vi "Interpret Driver Controls.vi"() -> ()   [LabVIEW 2018]
uses:
  SubSystems/Controllers/Manipulator Controlller/Manipulator Controller Global.vi
  SubSystems/Lift/Lift Global.vi
  SubSystems/Controllers/Driver Controller/Driver Controller Global.vi
  SubSystems/Cargo Intake/Cargo Intake Global.vi
  SubSystems/Drive Train/Drive Train Global.vi
  SubSystems/Hatch Panel Intake/Hatch Panel Intake Global.vi
panel:
  in  "y":dbl=0.6 format="%#_13g"
  in  "Y Slower":dbl=0.65
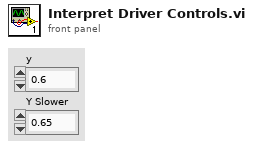
[diagram p1: front panel]
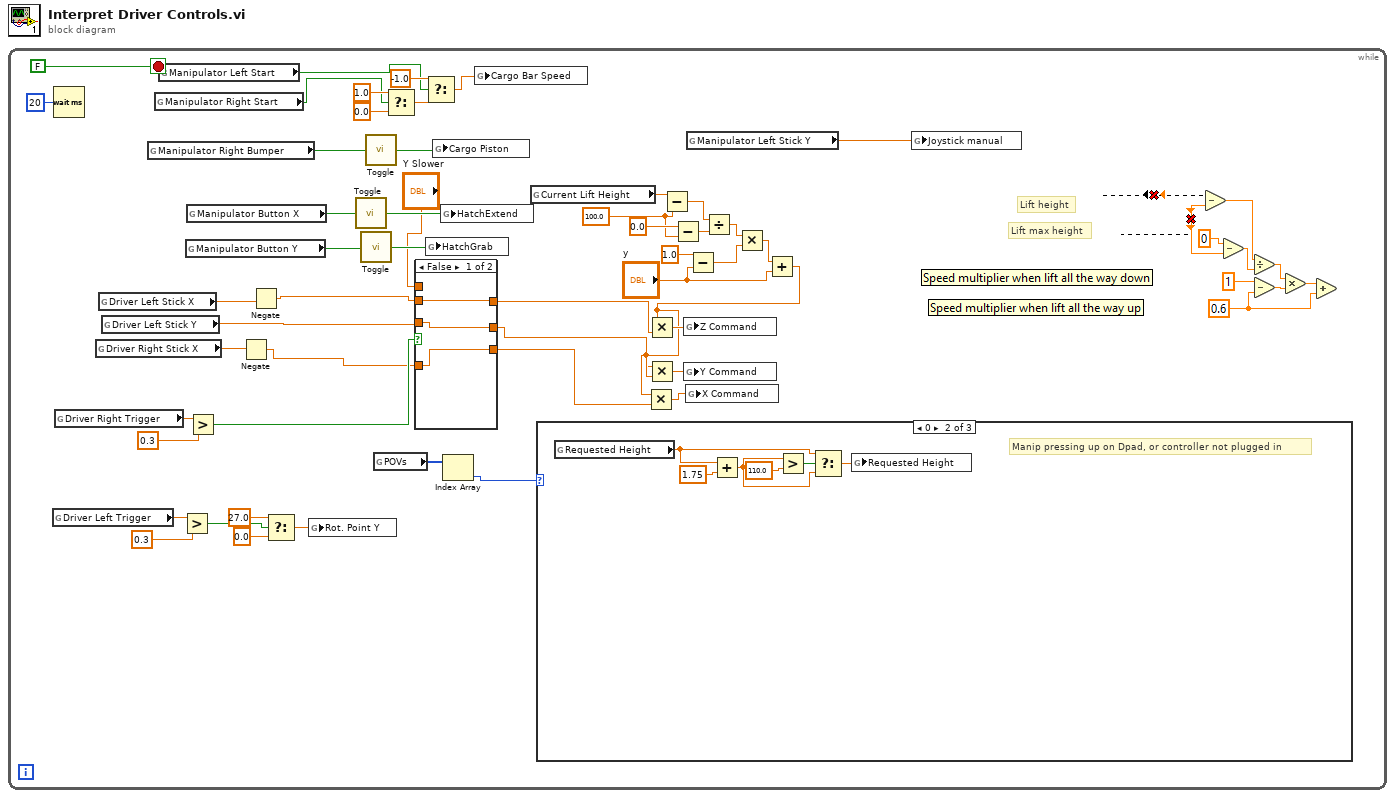
[diagram p0: block diagram]
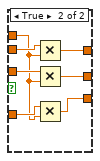
[diagram p2: hidden frame]
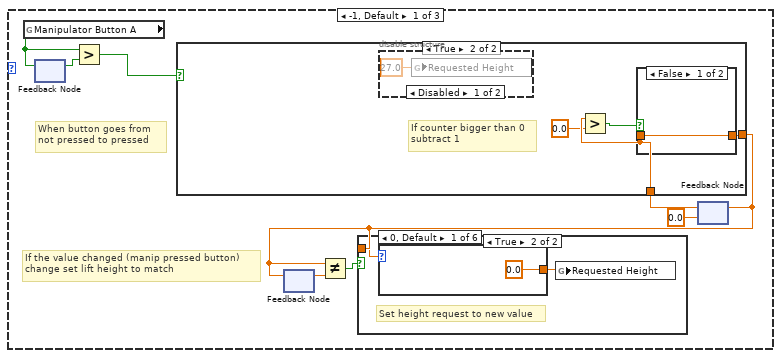
[diagram p3: hidden frame]
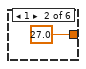
[diagram p5: hidden frame]
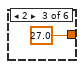
[diagram p6: hidden frame]
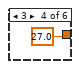
[diagram p7: hidden frame]
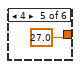
[diagram p8: hidden frame]
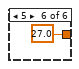
[diagram p9: hidden frame]
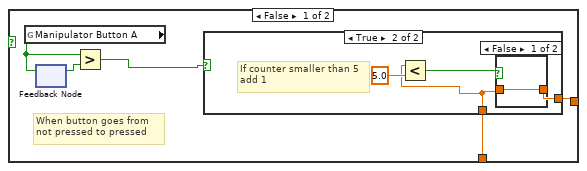
[diagram p10: hidden frame]
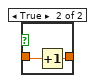
[diagram p12: hidden frame]
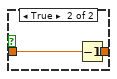
[diagram p13: hidden frame]
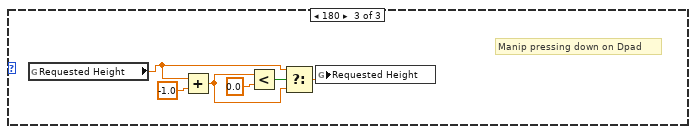
[diagram p15: hidden frame]
diagram:
  n1 = while {
    stop <- FALSE stop-if-true
    w10 = 100.0 ("y")
    # "Lift max height"
    # "Lift height"
    n2 = global read "Driver Controller Global.vi" "Driver Left Trigger"() -> (w5:dbl)
    n3 = Wait (ms)(milliseconds to wait=u32 20) -> ()  [unwired: 1 out]
    n4 = global read "Driver Controller Global.vi" "Driver Right Trigger"() -> (w32:dbl)
    n5 = global read "Driver Controller Global.vi" "Driver Right Stick X"() -> (w38:dbl)
    n6 = global read "Driver Controller Global.vi" "Driver Left Stick X"() -> (w39:dbl)
    n7 = global read "Driver Controller Global.vi" "Driver Left Stick Y"() -> (w8:dbl)
    n8 = global read "Manipulator Controller Global.vi" "Manipulator Right Bumper"() -> (w33:bool)
    n9 = global read "Manipulator Controller Global.vi" "Manipulator Right Start"() -> (w41:bool)
    n10 = global read "Manipulator Controller Global.vi" "Manipulator Left Start"() -> (w42:bool)
    n11 = Greater?(x=w5, y=0.3) -> (0:w3:bool)
    n12 = global read "Manipulator Controller Global.vi" "Manipulator Button Y"() -> (w37:bool)
    n13 = global read "Manipulator Controller Global.vi" "Manipulator Button X"() -> (w48:bool)
    n14 = Greater?(x=w32, y=0.3) -> (0:w28:bool)
    n15 = Negate(x=w38) -> (-x=w7:dbl)
    n16 = Negate(x=w39) -> (-x=w9:dbl)
    n17 = Select(t=27.0, s=w3, f=0.0) -> (s? t:f=w4:dbl)
    n18 = global write "Drive Train Global.vi" "Rot. Point Y"(w4) -> ()
    n19 = call "Toggle.vi"("Input"=w48) -> ("Output"=w47:bool)
    n20 = call "Toggle.vi"("Input"=w37) -> ("Output"=w36:bool)
    n21 = call "Toggle.vi"("Input"=w33) -> ("Output"=w34:bool)
    n22 = global read "Manipulator Controller Global.vi" "POVs"() -> (w30:i16[])
    n23 = Select(t=1.0, s=w41, f=0.0) -> (s? t:f=w46:dbl)
    n24 = case shown="False" w28 {
      tunnel: w9 -> [w53 w60]
      tunnel: "Y Slower" -> [_ w54]
      tunnel: [w53 w59] -> w23
      tunnel: [w52 w58] -> w22
      tunnel: [w51 w57] -> w21
      tunnel: w8 -> [w52 w56]
      tunnel: w7 -> [w51 w55]
      frame False {
      }
      frame True {
        n25 = Multiply(x=w60, y=w54) -> (x*y=w59:dbl)
        n26 = Multiply(x=w56, y=w54) -> (x*y=w58:dbl)
        n27 = Multiply(x=w55, y=w54) -> (x*y=w57:dbl)
      }
    }
    n28 = Select(t=-1.0, s=w42, f=w46) -> (s? t:f=w40:dbl)
    n29 = global write "Hatch Panel Intake Global.vi" "HatchGrab"(w36) -> ()
    n30 = global write "Cargo Intake Global.vi" "Cargo Piston"(w34) -> ()
    n31 = global write "Hatch Panel Intake Global.vi" "HatchExtend"(w47) -> ()
    n32 = Index Array(array=w30) -> (element=w29:i16)  [unwired: 1 in]
    n33 = global write "Cargo Intake Global.vi" "Cargo Bar Speed"(w40) -> ()
    n34 = global read "Lift Global.vi" "Current Lift Height"() -> (w20:dbl)
    n35 = case shown="0" w29 {
      frame -1, Default {
        # "If the value changed (manip pressed button)\nchange set lift height to match"
        # "When button goes from\nnot pressed to pressed"
        n36 = global read "Manipulator Controller Global.vi" "Manipulator Button A"() -> (w67:bool)
        n37 = feedback #1() -> (w68:bool)  [unwired: 1 in]
        n38 = feedback-in #1(w67) -> ()
        n39 = Greater?(x=w67, y=w68) -> (0:w61:bool)
        n40 = feedback #2() -> (w64:dbl)  [unwired: 1 in]
        n41 = feedback #3(0.0) -> (w66:dbl)
        n42 = case shown="True" w61 {
          tunnel: [w78 w93] -> w63
          tunnel: w66 -> [w79 w92]
          frame False {
            # "When button goes from\nnot pressed to pressed"
            n43 = global read "Manipulator Controller Global.vi" "Manipulator Button A"() -> (w81:bool)
            n44 = feedback #4() -> (w80:bool)  [unwired: 1 in]
            n45 = feedback-in #4(w81) -> ()
            n46 = Greater?(x=w81, y=w80) -> (0:w77:bool)
            n47 = case shown="True" w77 {
              tunnel: w79 -> [w82 w84]
              tunnel: [w82 w86] -> w78
              frame False {
              }
              frame True {
                # "If counter smaller than 5\nadd 1"
                n48 = Less?(x=w84, y=5.0) -> (x < y?=w83:bool)
                n49 = case shown="False" w83 {
                  tunnel: [w87 w89] -> w86
                  tunnel: w84 -> [w87 w88]
                  frame False {
                  }
                  frame True {
                    n50 = Increment(x=w88) -> (x+1=w89:dbl)
                  }
                }
              }
            }
          }
          frame True {
            # "If counter bigger than 0\nsubtract 1"
            n51 = disable-structure shown="Disabled" {
              frame Disabled {
                n52 = global write "Lift Global.vi" "Requested Height"(27.0 ("Requested Height")) -> ()
              }
              frame Enabled {
              }
            }
            n53 = Greater?(x=w92, y=0.0) -> (0:w91:bool)
            n54 = case shown="False" w91 {
              tunnel: [w94 w96] -> w93
              tunnel: w92 -> [w94 w95]
              frame False {
              }
              frame True {
                n55 = Decrement(x=w95) -> (x-1=w96:dbl)
              }
            }
          }
        }
        n56 = feedback-in #2(w63) -> ()
        n57 = Not Equal?(x=w63, y=w64) -> (x != y?=w62:bool)
        n58 = case shown="True" w62 {
          tunnel: w63 -> [_ w69]
          frame False {
            # "Manipulator didnt request change"
          }
          frame True {
            # "Set height request to new value"
            n59 = case shown="0, Default" w69 {
              tunnel: [0.0 ("Requested Height") 27.0 ("Requested Height") 27.0 ("Requested Height") 27.0 ("Requested Height") 27.0 ("Requested Height") 27.0 ("Requested Height")] -> w70
              frame 0, Default {
              }
              frame 1 {
              }
              frame 2 {
              }
              frame 3 {
              }
              frame 4 {
              }
              frame 5 {
              }
            }
            n60 = global write "Lift Global.vi" "Requested Height"(w70) -> ()
          }
        }
        n61 = feedback-in #3(w63) -> ()
      }
      frame 0 {
        # "Manip pressing up on Dpad, or controller not plugged in"
        n62 = global read "Lift Global.vi" "Requested Height"() -> (w99:dbl)
        n63 = Add(x=w99, y=1.75) -> (x+y=w98:dbl)
        n64 = Greater?(x=w98, y=110.0) -> (0:w100:bool)
        n65 = Select(t=w99, s=w100, f=w98) -> (s? t:f=w101:dbl)
        n66 = global write "Lift Global.vi" "Requested Height"(w101) -> ()
      }
      frame 180 {
        # "Manip pressing down on Dpad"
        n67 = global read "Lift Global.vi" "Requested Height"() -> (w104:dbl)
        n68 = Add(x=w104, y=-1.0) -> (x+y=w106:dbl)
        n69 = Less?(x=w106, y=0.0) -> (x < y?=w107:bool)
        n70 = Select(t=w104, s=w107, f=w106) -> (s? t:f=w105:dbl)
        n71 = global write "Lift Global.vi" "Requested Height"(w105) -> ()
      }
    }
    n72 = Subtract(x=w20, y=w10) -> (x-y=w19:dbl)
    n73 = Subtract(x=0.0 ("y"), y=w10) -> (x-y=w18:dbl)
    n74 = global read "Manipulator Controller Global.vi" "Manipulator Left Stick Y"() -> (w35:dbl)
    n75 = Subtract(x=1.0 ("y"), y="y") -> (x-y=w15:dbl)
    n76 = Divide(x=w19, y=w18) -> (x/y=w16:dbl)
    n77 = Multiply(x=w16, y=w15) -> (x*y=w14:dbl)
    n78 = Add(x=w14, y="y") -> (x+y=w12:dbl)
    n79 = Multiply(x=w12, y=w21) -> (x*y=w24:dbl)
    n80 = Multiply(x=w12, y=w23) -> (x*y=w26:dbl)
    n81 = Multiply(x=w12, y=w22) -> (x*y=w25:dbl)
    n82 = global write "Drive Train Global.vi" "Z Command"(w26) -> ()
    n83 = global write "Drive Train Global.vi" "Y Command"(w25) -> ()
    n84 = global write "Drive Train Global.vi" "X Command"(w24) -> ()
    n85 = global write "Lift Global.vi" "Joystick manual"(w35) -> ()
  }
